vi "Checks_Names Uniqueness.vi"(8 "error in (no error)":errorcluster, 11 "DMA":T1) -> (0 "error out":errorcluster)   [LabVIEW 2020, in "RefMem DMA System Explorer.lvlib"]
doc: "This VI checks that, for a given DMA Block, all Channels name are unique."
uses:
  RefMem DMA System Explorer.lvlib
  <userlib>/_OpenG.lib/array/array.llb/Remove Duplicates from 1D Array (String)__ogtk.vi
  controls/Typedef_DMA Instance.ctl
  controls/Typedef_Channel Settings.ctl
  controls/Data Channel Type.ctl
  controls/Typedef_DMA Block Settings.ctl
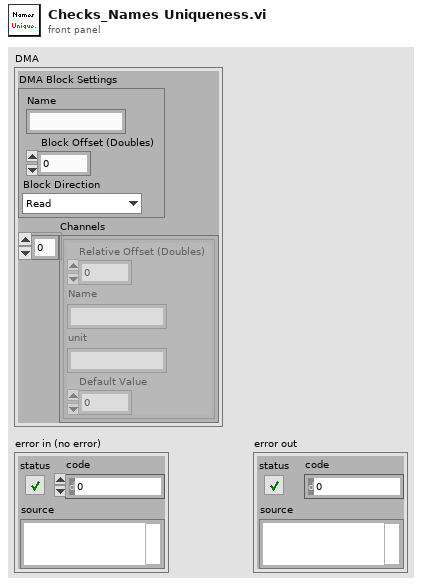
[diagram p1: front panel]
types:
  T1 = typedef "RefMem DMA System Explorer.lvlib/Typedef_DMA Instance.ctl" = cluster{"DMA Block Settings":T2, "Channels":T4[]}
  T2 = typedef "RefMem DMA System Explorer.lvlib/Typedef_DMA Block Settings.ctl" = cluster{"Name":string, " Block Offset (Doubles)":u32, "Block Direction":T3}
  T3 = typedef "RefMem DMA System Explorer.lvlib/Data Channel Type.ctl" = enum16{"Read", "Write"}
  T4 = typedef "RefMem DMA System Explorer.lvlib/Typedef_Channel Settings.ctl" = cluster{"Relative Offset (Doubles)":u32, "Name":string, "unit":string, "Default Value":dbl}
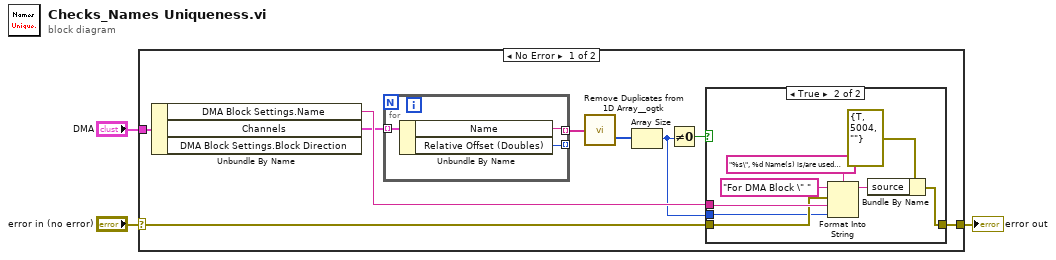
[diagram p0: block diagram]
diagram:
  n1 = case shown="No Error" "error in (no error)" {
    selector: "error in (no error)" -> [w4 w25]
    tunnel: [w11 w25] -> w3
    tunnel: "DMA" -> [w5 _]
    frame No Error {
      n2 = Unbundle By Name(w5) -> ("DMA Block Settings.Name"=w12:string, "Channels"=w6:T4[])  [unwired: 1 out]
      n3 = for {
        tunnel: w6 -> [w23] mode=indexing
        tunnel: [w24] -> w7 mode=indexing
        tunnel: [w22] -> _ mode=indexing
        n4 = Unbundle By Name(w23) -> ("Name"=w24:string, "Relative Offset (Doubles)"=w22:u32)
      }
      n5 = call-poly <userlib>:"Remove Duplicates from 1D Array__ogtk.vi"("Input Array"=w7) -> ("indices of removed elements"=w8:i32[])  [unwired: 1 out]
      n6 = Array Size(array=w8) -> (size(s)=w10:i32)
      n7 = Not Equal To 0?(x=w10) -> (x != 0?=w9:bool)
      n8 = case shown="True" w9 {
        tunnel: w4 -> [w13 w17]
        tunnel: [w13 w19] -> w11
        tunnel: w12 -> [_ w18]
        tunnel: w10 -> [_ w16]
        frame False {
        }
        frame True {
          n9 = Format Into String(format string="%s\", %d Name(s) is/are used multiple times. Within a DMA Block, each Channel Name must be unique.", initial string="For DMA Block \" ", error in=w17, w18, w16) -> (resulting string=w20:string)  [unwired: 1 out]
          n10 = Bundle By Name(cluster=errorcluster {"status"=TRUE, "code"=5004, "source"=""} ("error IO"), "source"=w20) -> (w19:errorcluster)
        }
      }
    }
    frame Error {
    }
  }
  "error out" <- w3
